vi "Tag-Remove Tag.vi"(8 "error in (no error)":errorcluster, 10 "Tag Name":string, 11 "Generic in":refnum<class "Generic.lvclass">) -> (0 "error out":errorcluster, 1 "Old Value":variant, 2 "Tag:Remove Tag":bool, 3 "Generic out":refnum<class "Generic.lvclass">)   [LabVIEW 2015, in "Generic.lvclass"]
doc: "Removes the specified tag. Returns FALSE if LabVIEW did not remove the tag.\n\nQControl Class wrapper around the <b>Generic : Tag:Remove Tag Method</b>.\n<b> </b> <b> </b>\n©2016 Q Software Innovations, LLC (QSI)\nwritten by Quentin Alldredge\nproduced in LabVIEW 2015\n\nsupport@qsoftwareinnovations.com\nwww.qsoftwareinnovations.com\n\nAll rights reserved.\n\nRedistribution and use in source and binary forms, with or without modification, are permitted provided that the following conditions are met:\n\n * Redistributions of source code must retain the above copyright notice, this list of conditions and the following disclaimer.\n * Redistributions in binary form must reproduce the above copyright notice, this list of conditions and the following disclaimer in the documentation and/or other materials provided with the distribution.\n * Neither the name of Q Software Innovations, LLC. nor the names of its contributors may be used to endorse or promote products derived from this software without specific prior written permission.\n\nTHIS SOFTWARE IS PROVIDED BY THE COPYRIGHT HOLDERS AND CONTRIBUTORS \"AS IS\" AND ANY EXPRESS OR IMPLIED WARRANTIES, INCLUDING, BUT NOT LIMITED TO, THE IMPLIED WARRANTIES OF MERCHANTABILITY AND FITNESS FOR A PARTICULAR PURPOSE ARE DISCLAIMED. IN NO EVENT SHALL THE COPYRIGHT OWNER OR CONTRIBUTORS BE LIABLE FOR ANY DIRECT, INDIRECT, INCIDENTAL, SPECIAL, EXEMPLARY, OR CONSEQUENTIAL DAMAGES (INCLUDING, BUT NOT LIMITED TO, PROCUREMENT OF SUBSTITUTE GOODS OR SERVICES; LOSS OF USE, DATA, OR PROFITS; OR BUSINESS INTERRUPTION) HOWEVER CAUSED AND ON ANY THEORY OF LIABILITY, WHETHER IN CONTRACT, STRICT LIABILITY, OR TORT (INCLUDING NEGLIGENCE OR OTHERWISE) ARISING IN ANY WAY OUT OF THE USE OF THIS SOFTWARE, EVEN IF ADVISED OF THE POSSIBILITY OF SUCH DAMAGE."
uses:
  Generic.lvclass
  Generic.lvclass/Generic.ctl
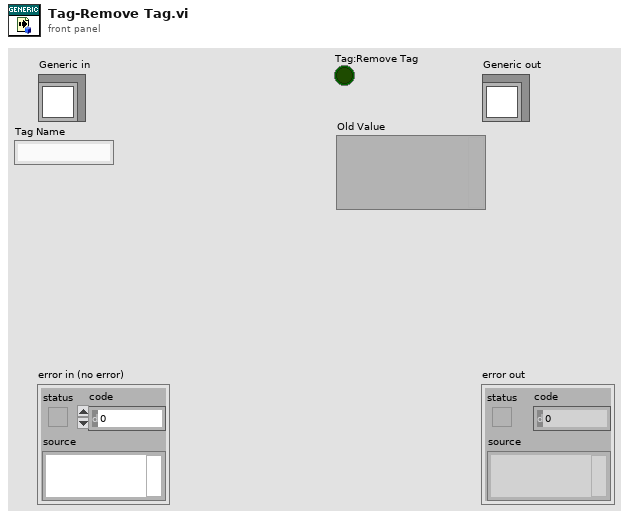
[diagram p1: front panel]
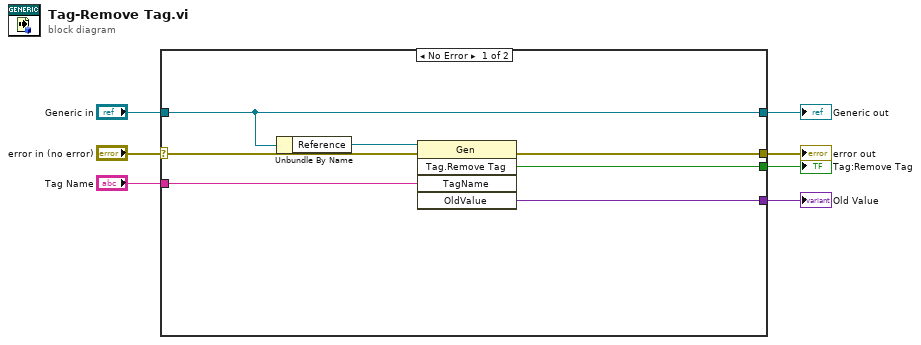
[diagram p0: block diagram]
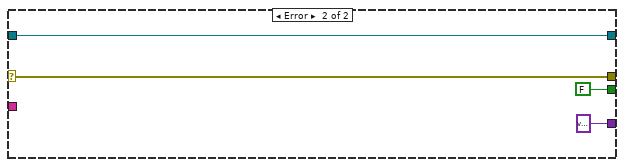
[diagram p2: hidden frame]
diagram:
  n1 = case shown="No Error" "error in (no error)" {
    selector: "error in (no error)" -> [w14 w18]
    tunnel: [w13 w18] -> w6
    tunnel: [w12 w17] -> w4
    tunnel: "Generic in" -> [w12 w17]
    tunnel: "Tag Name" -> [w10 _]
    tunnel: [w9 FALSE ("RemoveTag")] -> w2
    tunnel: [w8 variant ("OldValue")] -> w1
    frame No Error {
      n2 = Unbundle By Name(w12) -> ("Reference"=w11:refnum<vi>)
      n3 = invoke class="Gen" method="Tag.Remove Tag"(reference=w11, error in=w14, "TagName"=w10) -> (error out=w13:errorcluster, "RemoveTag"=w9:bool, "OldValue"=w8:variant)  [unwired: 2 in, 2 out]
    }
    frame Error {
    }
  }
  "error out" <- w6
  "Generic out" <- w4
  "Tag:Remove Tag" <- w2
  "Old Value" <- w1
